vi "2.2.vi"(10 "Numeric":dbl) -> (2 "Numeric 2":dbl)   [LabVIEW 2013]
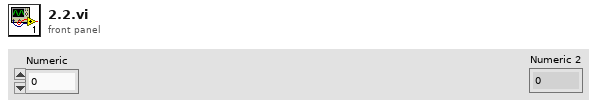
[diagram p1: front panel]
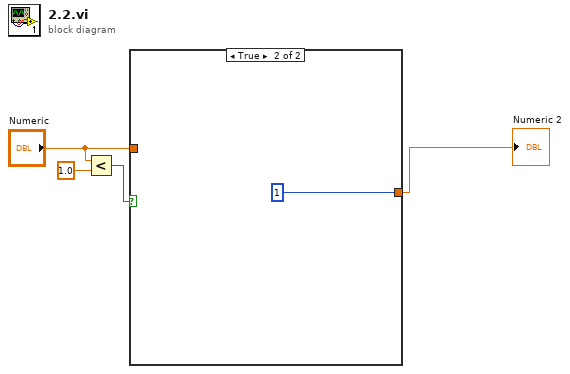
[diagram p0: block diagram]
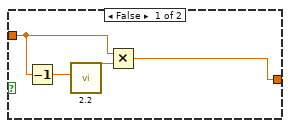
[diagram p2: hidden frame]
diagram:
  n1 = Less?(x="Numeric", y=1.0) -> (x < y?=w3:bool)
  n2 = case shown="True" w3 {
    tunnel: [w8 1] -> w1
    tunnel: "Numeric" -> [w6 _]
    frame False {
      n3 = Decrement(x=w6) -> (x-1=w5:dbl)
      n4 = call "2.2.vi"("Numeric"=w5) -> ("Numeric 2"=w7:dbl)  [unwired: 10 in]
      n5 = Multiply(x=w6, y=w7) -> (x*y=w8:dbl)
    }
    frame True {
    }
  }
  "Numeric 2" <- w1
